vi "簇函数.vi"() -> ()   [LabVIEW 2018]
panel:
  out "数组 2":cluster{"姓名":string, "学号":string}[](array[cluster])
  in  "数组":T1(array[cluster])
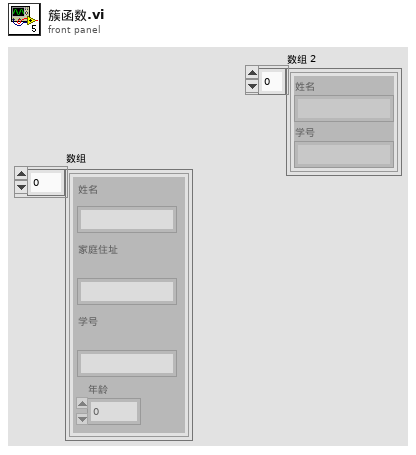
[diagram p1: front panel]
types:
  T1 = cluster{"\n姓名":string, "家庭住址":string, "学号":string, "年龄":dbl}[]
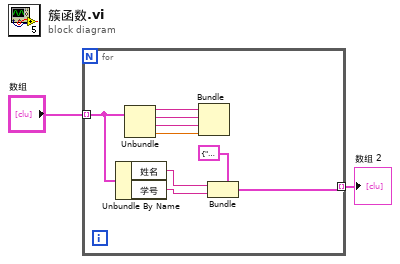
[diagram p0: block diagram]
diagram:
  n1 = for {
    tunnel: "数组" -> [w11] mode=indexing
    tunnel: [w7] -> w1 mode=indexing
    n2 = Unbundle By Name(w11) -> ("姓名"=w9:string, "学号"=w8:string)
    n3 = Unbundle(w11) -> ("姓名"=w6:string, "家庭住址"=w5:string, "学号"=w4:string, "年龄"=w3:dbl)
    n4 = Bundle("姓名"=w6, "家庭住址"=w5, "学号"=w4, "年龄"=w3) -> ()  [unwired: 1 in, 1 out]
    n5 = Bundle(cluster=cluster{"姓名":string, "学号":string} {"姓名"="", "学号"=""}, "姓名"=w9, "学号"=w8) -> (w7:cluster{"姓名":string, "学号":string})
  }
  "数组 2" <- w1
